vi "Mapping v10.6.0.vi"(5 "Simulate Spectra":bool, 7 "Simulate Drive":bool) -> ()   [LabVIEW 2010]
uses:
  TypeDefs/Mapping Spectra Params.ctl
  TypeDefs/Mapping Drive Params v10.6.0.ctl
  NPC3SG/TypeDefs/NPC3SG Set Positions.ctl
  NPC3SG/TypeDefs/NPC3SG Current Values.ctl
  iHR550/TypeDefs/iHR Current Values.ctl
  ITC503/TypeDefs/ITC503 Current Values.ctl
  TypeDefs/Mapping Input Parameters v10.6.0.ctl
  Symphony/TypeDefs/Symphony Area Format.ctl
  <vilib>/Utility/miscctls.llb/LVPointTypeDef.ctl
  Global Variables.vi
panel:
  in  "Input Parameters":T1={"Drive Connection Port"="", "ITC503 Current Values"={"ITC503 Heater"=0.0, "ITC503 Temperature"=0.0, "ITC503 P"=0.0, "ITC503 I"=0.0, "ITC503 D"=0.0, "ITC503 Setpoint"=0.0, "ITC503 Gradient"=0.0, "ITC503 Heater Auto"=FALSE, "ITC503 PID Auto"=FALSE}, "Wavelengths (nm)"=[], "Drive Current Values"={"Drive X Position"=0.0, "Drive Y Position"=0.0, "Drive Z Position"=0.0}, "iHR Current Values"={"iHR 550 Front Entrance"=0.0, "iHR550 Side Exit"=0.0, "iHR550 Wavelength"=897.9988, "iHR550 Exit Mirror"=2, "iHR550 Grating"="1", "Grating Index"=1}, "Spectra Settings"={"Integration Time"=1.0, "Repetitions"=1, "Mapping Spectra"=TRUE}, "CCD3500 Temperature"=0.0, "Simulate Drive"=FALSE, "Simulate Spectra"=FALSE, "JYCCDLib.IJYCCDReqd"=refnum, "CCD Area"={"XStart"=1, "YStart"=1, "XStop"=2048, "YStop"=512, "XBin"=1, "YBin"=1}, "CCD Gain"=1, "CCD ADC"=0} {"CCD ADC" items=["20 kHz       ", " 1 MHz       ", " 1 MHz Ultra ", "500 kHz Wrap"]; "CCD Gain" items=["High Light", "Best Dynamic Range", "High Sensitivity"]; "ITC503 Current Values"."ITC503 Gradient" format="%.2f"; "ITC503 Current Values"."ITC503 Setpoint" min=-273.0 max=300000.0 step=0.0001 format="%.1f"; "ITC503 Current Values"."ITC503 I" format="%_1f"; "ITC503 Current Values"."ITC503 P" format="%_1f"; "ITC503 Current Values"."ITC503 Temperature" min=0.0 max=1645.0 step=1e-05 format="%.2f"; "ITC503 Current Values"."ITC503 Heater" min=0.0 max=100.0 step=0.01 scale=0.0..100.0; "Drive Current Values"."Drive Z Position" min=-273.0 max=300000.0 step=0.0001 format="%.3f"; "Drive Current Values"."Drive Y Position" min=-273.0 max=300000.0 step=0.0001 format="%.3f"; "Drive Current Values"."Drive X Position" min=-273.0 max=300000.0 step=0.0001 format="%.3f"; "iHR Current Values"."iHR550 Exit Mirror" items=["EntranceMirror", "ExitMirror", "Front", "Side"]; "Spectra Settings"."Repetitions" min=1 max=100 step=1; "Spectra Settings"."Integration Time" min=0.5 max=6000.0 step=1.0 format="%.1f"}
  out "JYCCDLib.IJYCCDReqd":refnum<k7>
  out "AutoClose":bool
  out "ITC503 Temperature":dbl caption="Sample (K)" min=10.0 max=160.0 step=0.1 format="%.3f"
  out "CCD3500 Temperature":dbl caption="CCD (°C)" min=10.0 max=160.0 step=0.1 format="%.1f"
  in  "CCD Current Rep.":string="0/0"
  in  "Pause":bool
  out "Current Position":T3 {"Drive Z Position" min=-273.0 max=300000.0 step=0.0001 format="%.3f"; "Drive Y Position" min=-273.0 max=300000.0 step=0.0001 format="%.3f"; "Drive X Position" min=-273.0 max=300000.0 step=0.0001 format="%.3f"}
  out "Target Position":T7={"Drive X Set"=10.0, "Drive Y Set"=10.0, "Drive Z Set"=10.0} {"Drive X Set" min=10.0 max=160.0 step=0.1 format="%.3f"; "Drive Z Set" min=10.0 max=160.0 step=0.1 format="%.3f"; "Drive Y Set" min=10.0 max=160.0 step=0.1 format="%.3f"}
  out "Progress":u8(slide) max=10 scale=0.0..100.0
  out "Objective Running":bool caption="Obj."
  out "CCD Running":bool caption="CCD"
  in  "Save Map":bool
  in  "Spectra Params":T5={"Integration Time"=10.0, "Repetitions"=10, "Mapping Spectra"=TRUE} {"Repetitions" min=1 max=100 step=1; "Integration Time" min=0.5 max=6000.0 step=1.0 format="%.1f"}
  in  "Drive Settings":refnum<visa-resource-name>
  in  "Z Position":dbl caption="Z (µm)" min=0.0 max=100.0 step=0.1 format="%.1f"
  in  "Mapping Params":T8={"X Start Position"=0.0, "X Stop Position"=10.0, "Y Start Position"=0.0, "Y Stop Position"=10.0, "Step Size"=1.0} {"Step Size" min=0.005 max=20.0 step=0.005 format="%.3f"; "Y Stop Position" min=0.0 max=140.0 step=0.005 format="%.3f"; "Y Start Position" min=0.0 max=140.0 step=0.005 format="%.3f"; "X Stop Position" min=0.0 max=140.0 step=0.005 format="%.3f"; "X Start Position" min=0.0 max=140.0 step=0.005 format="%.3f"}
  in  "Exit":bool
  out "Measuring":bool
  in  "Start":bool
  out "Filename":string
  out "Full Data":dbl[][](array[numeric])
  out "Live Data":dbl[][](array[numeric])
  in  "ITC503 Current Values":T2 {"ITC503 Gradient" format="%.2f"; "ITC503 Setpoint" min=-273.0 max=300000.0 step=0.0001 format="%.1f"; "ITC503 I" format="%_1f"; "ITC503 P" format="%_1f"; "ITC503 Temperature" min=0.0 max=1645.0 step=1e-05 format="%.2f"; "ITC503 Heater" min=0.0 max=100.0 step=0.01 scale=0.0..100.0}
  in  "iHR Current Values":T4={"iHR 550 Front Entrance"=0.0, "iHR550 Side Exit"=0.0, "iHR550 Wavelength"=897.9988, "iHR550 Exit Mirror"=2, "iHR550 Grating"="1", "Grating Index"=1} {"iHR550 Exit Mirror" items=["EntranceMirror", "ExitMirror", "Front", "Side"]}
  in  "Wavelengths (nm)":dbl[](array[numeric])
  # "Status"
  # "Active"
  # "Target"
  # "Current"
  # "Parameters"
  # "Spectral"
  # "Spectral / Video Mapping"
  # "Mapping"
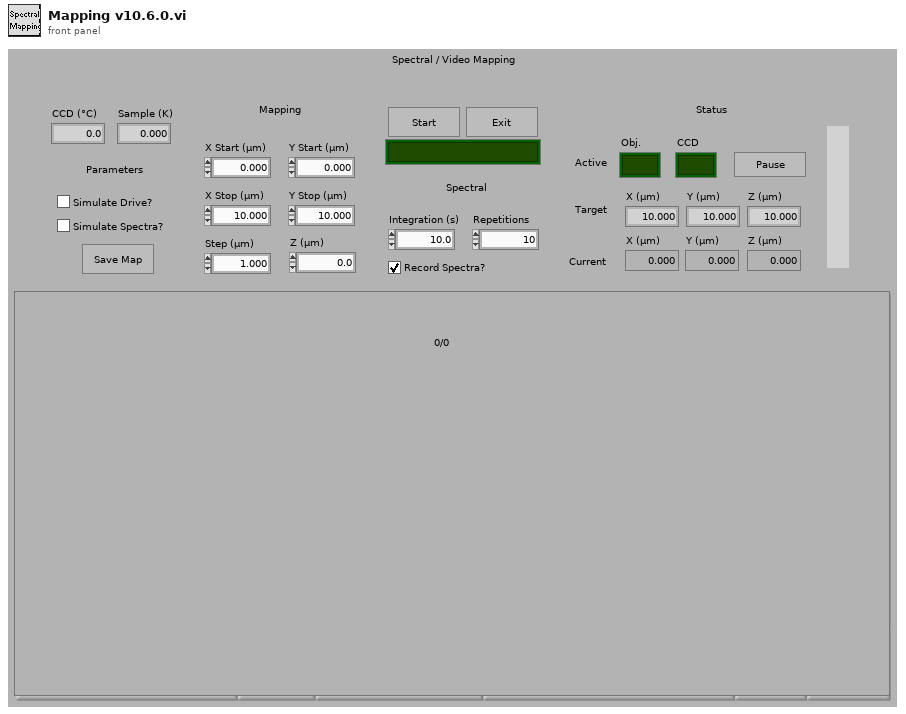
[diagram p1: front panel]
types:
  T1 = typedef "Mapping Input Parameters v10.6.0.ctl" = cluster{"Drive Connection Port":refnum<visa-resource-name>, "ITC503 Current Values":T2, "Wavelengths (nm)":dbl[], "Drive Current Values":T3, "iHR Current Values":T4, "Spectra Settings":T5, "CCD3500 Temperature":dbl, "Simulate Drive":bool, "Simulate Spectra":bool, "JYCCDLib.IJYCCDReqd":refnum<k7>, "CCD Area":T6, "CCD Gain":u16, "CCD ADC":u16}
  T2 = typedef "ITC503 Current Values.ctl" = cluster{"ITC503 Heater":dbl, "ITC503 Temperature":dbl, "ITC503 P":dbl, "ITC503 I":dbl, "ITC503 D":dbl, "ITC503 Setpoint":dbl, "ITC503 Gradient":dbl, "ITC503 Heater Auto":bool, "ITC503 PID Auto":bool}
  T3 = typedef "NPC3SG Current Values.ctl" = cluster{"Drive X Position":dbl, "Drive Y Position":dbl, "Drive Z Position":dbl}
  T4 = typedef "iHR Current Values.ctl" = cluster{"iHR 550 Front Entrance":dbl, "iHR550 Side Exit":dbl, "iHR550 Wavelength":dbl, "iHR550 Exit Mirror":i32, "iHR550 Grating":string, "Grating Index":i32}
  T5 = typedef "Mapping Spectra Params.ctl" = cluster{"Integration Time":dbl, "Repetitions":u16, "Mapping Spectra":bool}
  T6 = typedef "Symphony Area Format.ctl" = cluster{"XStart":i32, "YStart":i32, "XStop":i32, "YStop":i32, "XBin":i32, "YBin":i32}
  T7 = typedef "NPC3SG Set Positions.ctl" = cluster{"Drive X Set":dbl, "Drive Y Set":dbl, "Drive Z Set":dbl}
  T8 = typedef "Mapping Drive Params v10.6.0.ctl" = cluster{"X Start Position":dbl, "X Stop Position":dbl, "Y Start Position":dbl, "Y Stop Position":dbl, "Step Size":dbl}
  T9 = typedef "LVPointTypeDef.ctl" = cluster{"Horizontal":i16, "Vertical":i16}
  T10 = cluster{"Intensities":dbl[], "Wavelengths":dbl[]}[]
  T11 = cluster{"Intensities":dbl[], "Wavelengths":dbl[]}
  T12 = enum32{"invalid app kind", "Development System", "Run Time System", "Student Edition", "Embedded LabVIEW", "Evaluation", "Custom"}
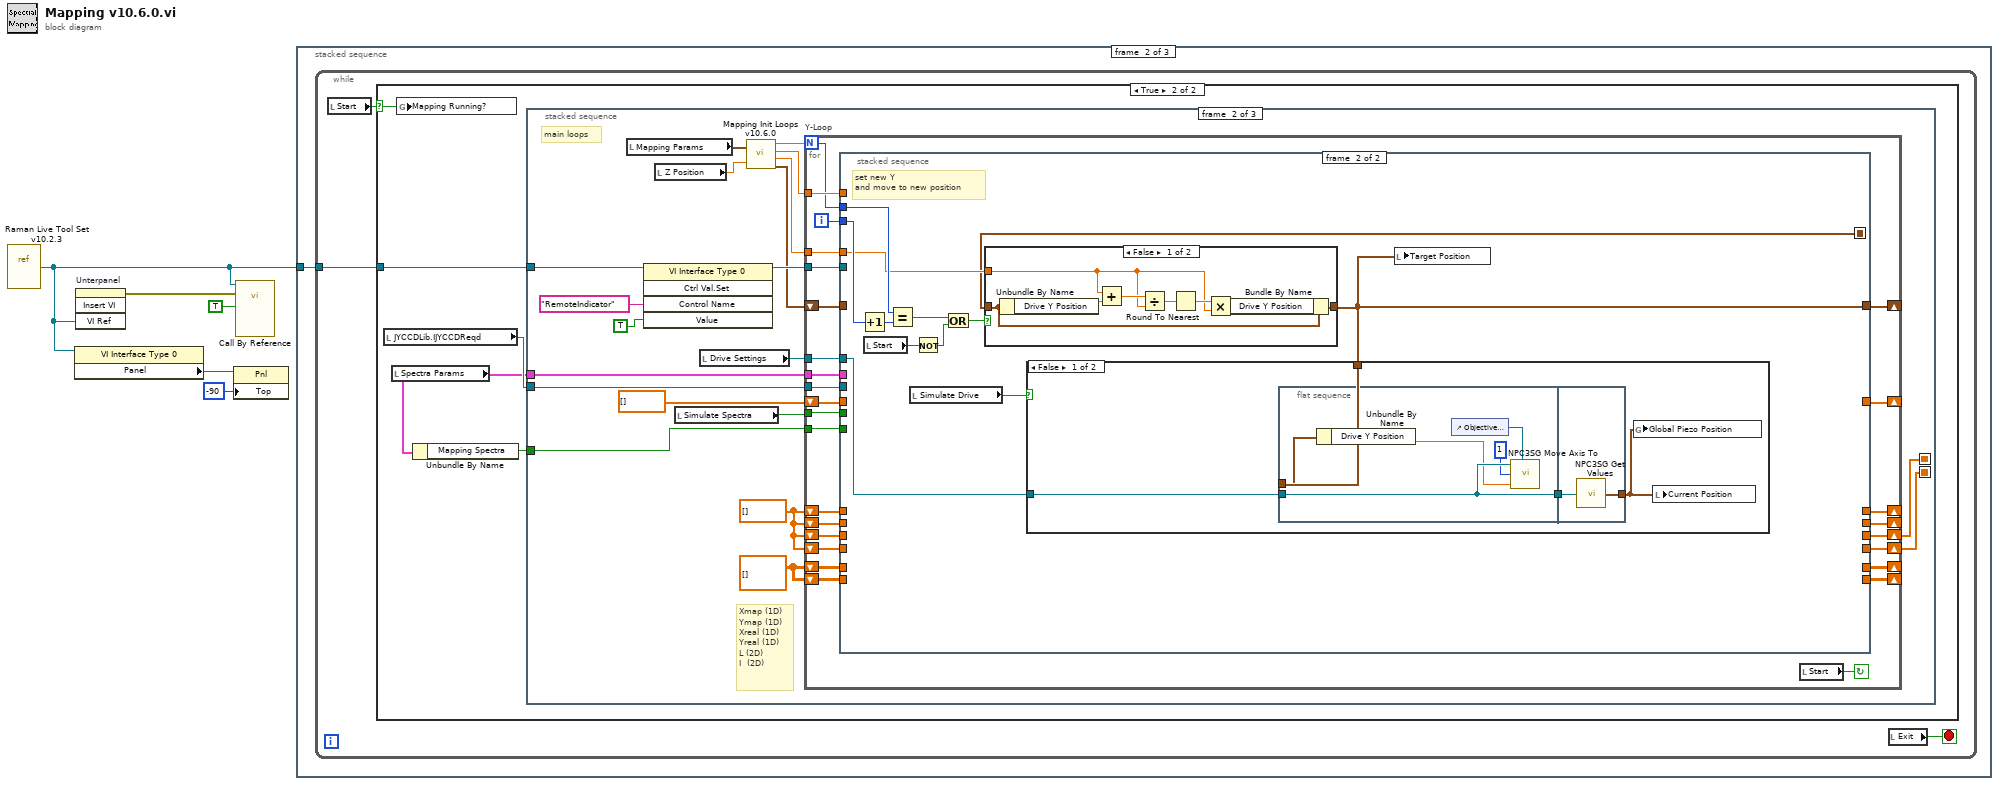
[diagram p0: block diagram]
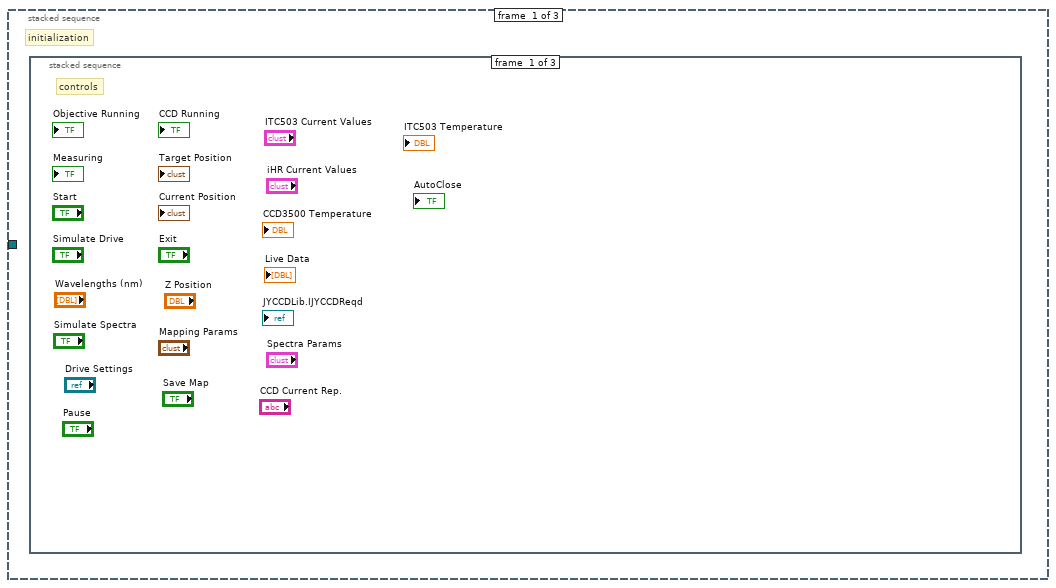
[diagram p2: hidden frame]
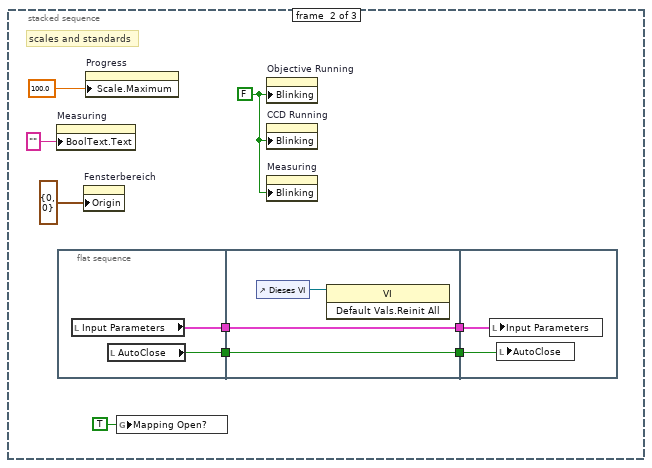
[diagram p3: hidden frame]
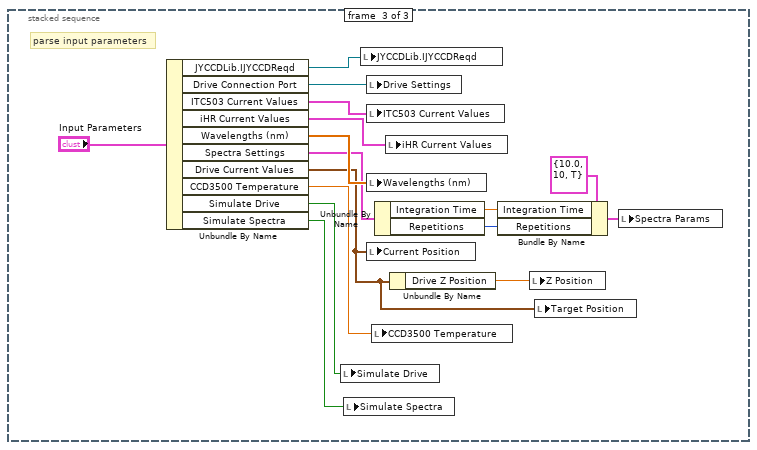
[diagram p4: hidden frame]
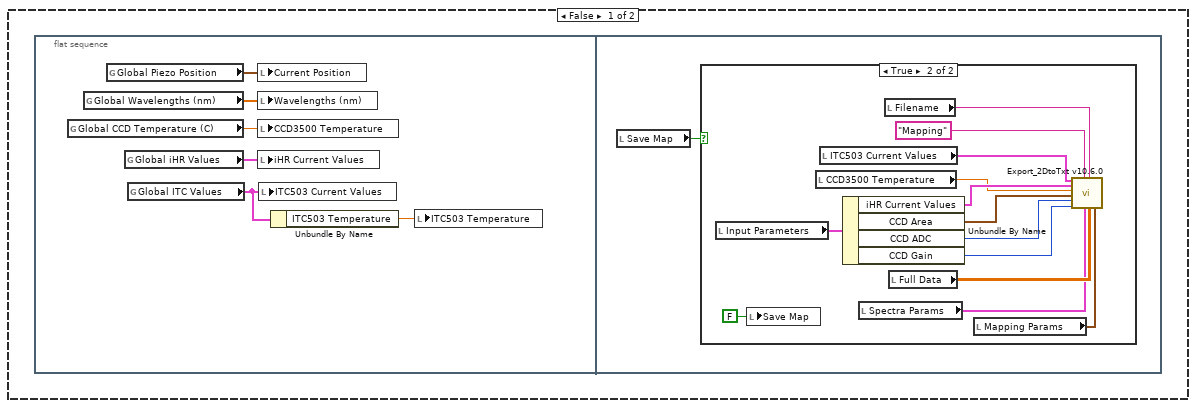
[diagram p5: hidden frame]
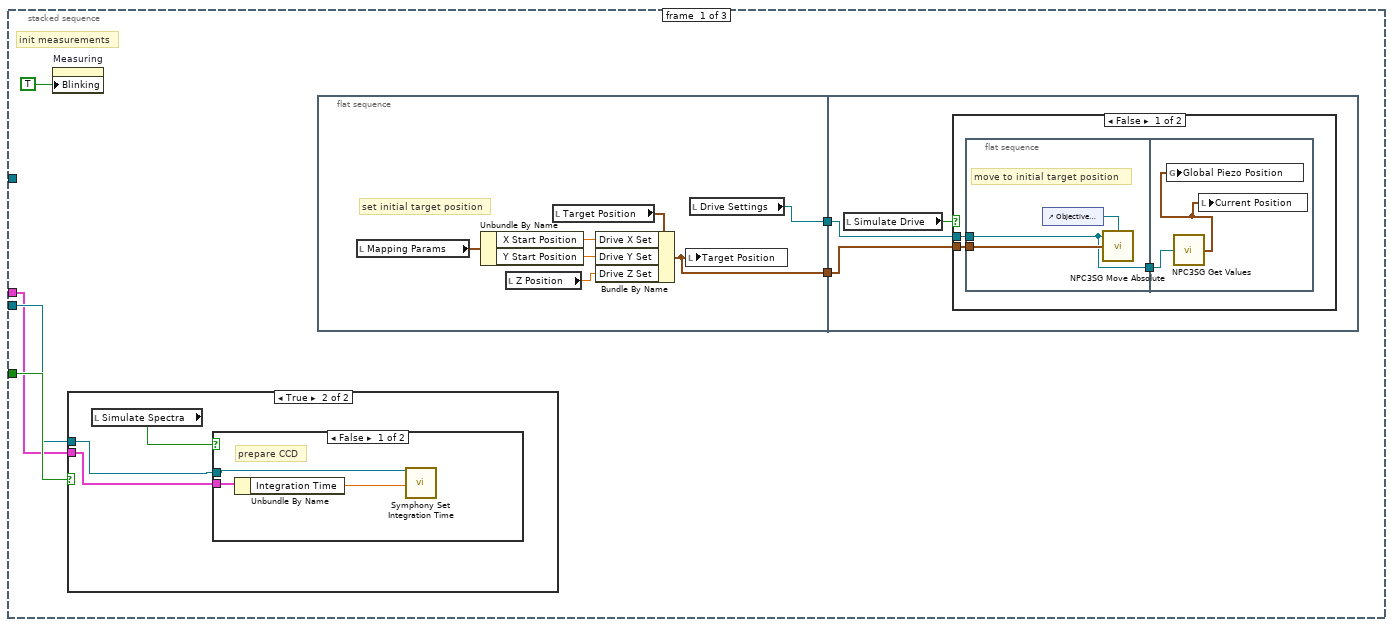
[diagram p7: hidden frame]
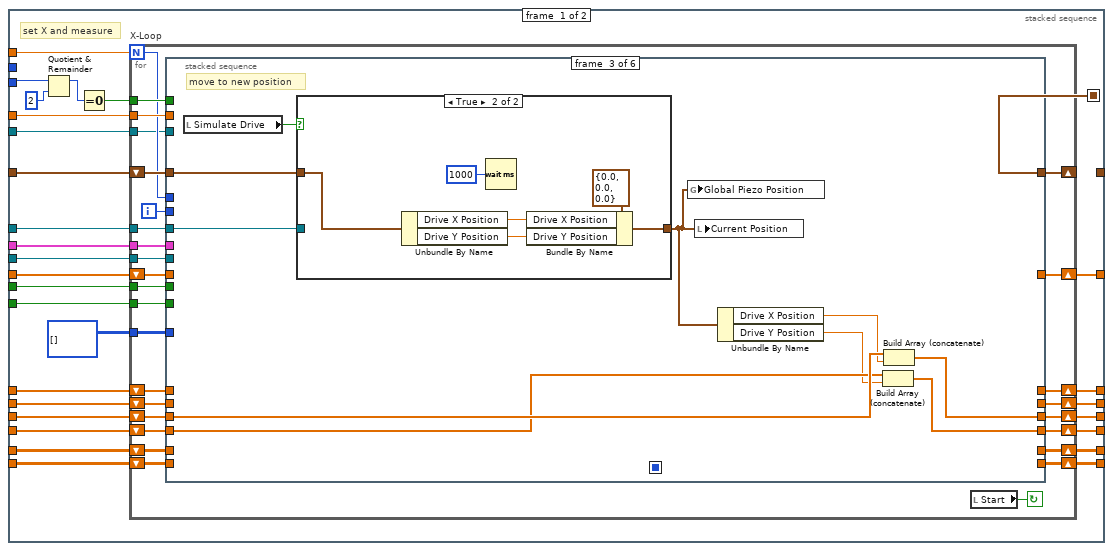
[diagram p11: hidden frame]
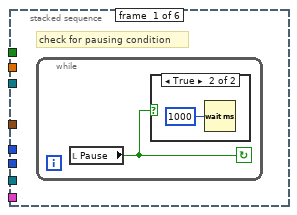
[diagram p12: hidden frame]
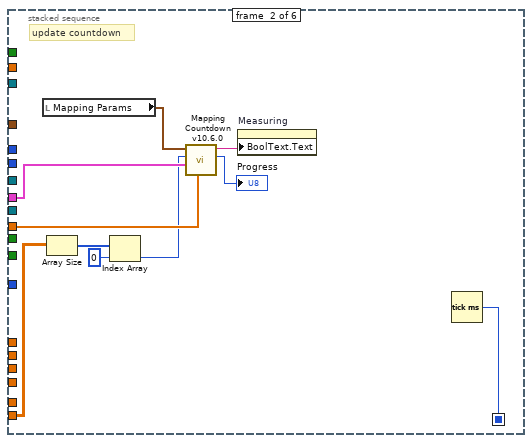
[diagram p14: hidden frame]
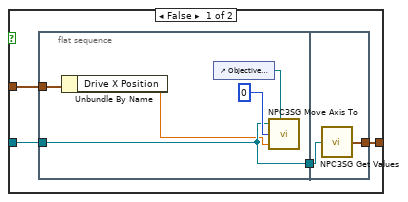
[diagram p15: hidden frame]
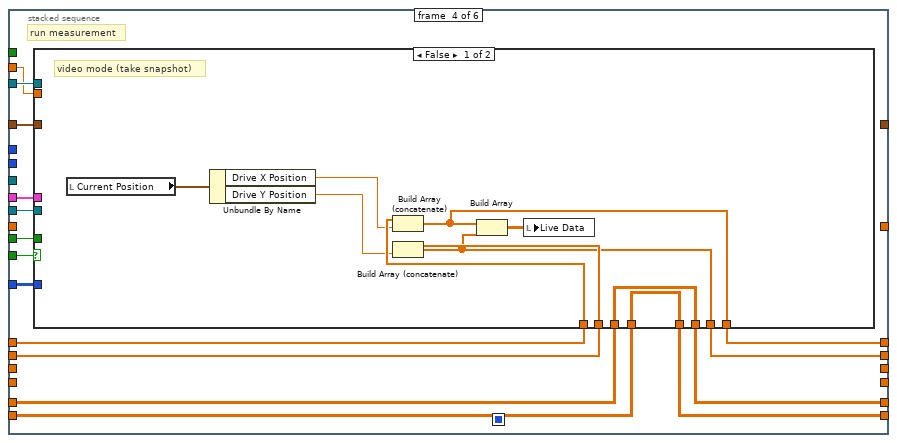
[diagram p16: hidden frame]
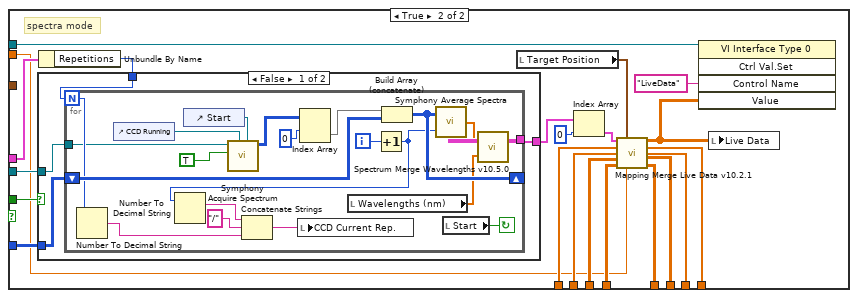
[diagram p17: hidden frame]
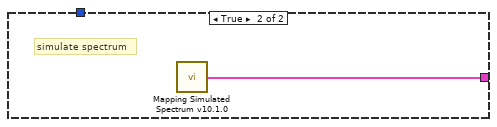
[diagram p18: hidden frame]
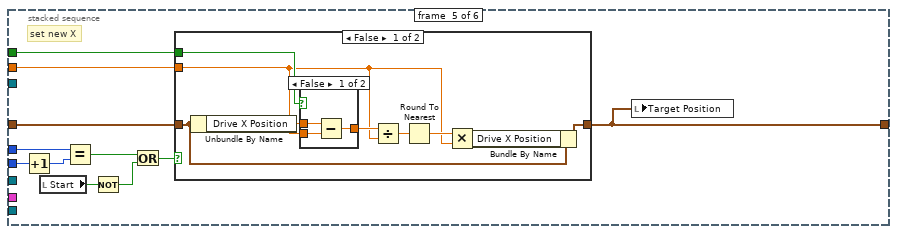
[diagram p19: hidden frame]
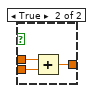
[diagram p20: hidden frame]
diagram:
  n1 = vi-ref "Raman Live Tool Set v10.2.3.vi"() -> (w3:refnum<vi>)
  n2 = property class="VI Interface Type 0"(reference=w3) -> ("Panel"=w2:refnum<vi>)  [unwired: 1 in, 2 out]
  n3 = invoke on="Unterpanel" class="Unterpanel" method="Insert VI"("VI Ref"=w3) -> (error out=w5:errorcluster)  [unwired: 3 in, 3 out]
  n4 = property class="Pnl"(reference=w2, "Top"=-90 ("Position:Oben")) -> ()  [unwired: 1 in, 2 out]
  n5 = call-by-ref "?"(reference=w3, error in=w5, "RemoteIndicator"=TRUE) -> ()  [unwired: 3 in, 2 out]
  n6 = stacked-sequence {
    tunnel: w3 -> [_ w38 w404]
    frame #0 {
      # "initialization"
      n7 = stacked-sequence {
        frame #0 {
          # "controls"
        }
        frame #1 {
          w12 = FALSE ("Blinkend")
          # "scales and standards"
          n8 = property on="Measuring" class="Bool (strict)"("BoolText.Text"="" ("Boolescher Text.Text")) -> ()  [unwired: 2 in, 2 out]
          n9 = flat-sequence {
            tunnel: [w16] -> w9
            tunnel: [w15] -> w6
            tunnel: [w18] -> w10
            tunnel: w9 -> [w18]
            tunnel: [w17] -> w7
            tunnel: w6 -> [w17]
            tunnel: w10 -> [w21]
            tunnel: w7 -> [w20]
            frame #0 {
              n10 = local read "Input Parameters"() -> (w16:T1)
              n11 = local read "AutoClose"() -> (w15:bool)
            }
            frame #1 {
              n12 = control-ref of="Dieses VI"() -> (w19:refnum<vi>)
              n13 = invoke class="VI" method="Default Vals.Reinit All"(reference=w19) -> ()  [unwired: 2 in, 3 out]
            }
            frame #2 {
              n14 = local write "Input Parameters"(w21) -> ()
              n15 = local write "AutoClose"(w20) -> ()
            }
          }
          n16 = property on="Fensterbereich" class="Pane"("Origin"=T9 {"Horizontal"=0, "Vertical"=0}) -> ()  [unwired: 2 in, 2 out]
          n17 = property on="Progress" class="Slide (strict)"("Scale.Maximum"=100.0 ("Skalierung.Bereich:Maximum")) -> ()  [unwired: 2 in, 2 out]
          n18 = global write "Global Variables.vi" "Mapping Open?"(TRUE ("Mapping Open?")) -> ()
          n19 = property on="Objective Running" class="Bool (strict)"("Blinking"=w12) -> ()  [unwired: 2 in, 2 out]
          n20 = property on="CCD Running" class="Bool (strict)"("Blinking"=w12) -> ()  [unwired: 2 in, 2 out]
          n21 = property on="Measuring" class="Bool (strict)"("Blinking"=w12) -> ()  [unwired: 2 in, 2 out]
        }
        frame #2 {
          # "parse input parameters"
          n22 = Unbundle By Name("Input Parameters") -> ("JYCCDLib.IJYCCDReqd"=w24:refnum<k7>, "Drive Connection Port"=w36:refnum<visa-resource-name>, "ITC503 Current Values"=w37:T2, "iHR Current Values"=w27:T4, "Wavelengths (nm)"=w35:dbl[], "Spectra Settings"=w33:T5, "Drive Current Values"=w22:T3, "CCD3500 Temperature"=w28:dbl, "Simulate Drive"=w26:bool, "Simulate Spectra"=w25:bool)
          n23 = local write "Simulate Drive"(w26) -> ()
          n24 = local write "Simulate Spectra"(w25) -> ()
          n25 = local write "JYCCDLib.IJYCCDReqd"(w24) -> ()
          n26 = local write "Drive Settings"(w36) -> ()
          n27 = local write "ITC503 Current Values"(w37) -> ()
          n28 = local write "Wavelengths (nm)"(w35) -> ()
          n29 = local write "Current Position"(w22) -> ()
          n30 = local write "CCD3500 Temperature"(w28) -> ()
          n31 = Unbundle By Name(w33) -> ("Integration Time"=w31:dbl, "Repetitions"=w30:u16)
          n32 = local write "iHR Current Values"(w27) -> ()
          n33 = Unbundle By Name(w22) -> ("Drive Z Position"=w34:dbl)
          n34 = Bundle By Name(cluster=T5 {"Integration Time"=10.0, "Repetitions"=10, "Mapping Spectra"=TRUE} ("Mapping Spectra Settings"), "Integration Time"=w31, "Repetitions"=w30) -> (w29:T5)
          n35 = local write "Z Position"(w34) -> ()
          n36 = local write "Target Position"(w22) -> ()
          n37 = local write "Spectra Params"(w29) -> ()
        }
      }
    }
    frame #1 {
      n38 = while {
        tunnel: w38 -> [w41]
        stop <- w40 stop-if-true
        n39 = local read "Start"() -> (w39:bool)
        n40 = case shown="True" w39 {
          selector: w39 -> [_ w62]
          tunnel: w41 -> [_ w66]
          frame False {
            n41 = flat-sequence {
              frame #0 {
                n42 = global read "Global Variables.vi" "Global CCD Temperature (C)"() -> (w47:dbl)
                n43 = global read "Global Variables.vi" "Global Wavelengths (nm)"() -> (w45:dbl[])
                n44 = global read "Global Variables.vi" "Global Piezo Position"() -> (w46:T3)
                n45 = global read "Global Variables.vi" "Global iHR Values"() -> (w44:T4)
                n46 = global read "Global Variables.vi" "Global ITC Values"() -> (w43:T2)
                n47 = local write "Current Position"(w46) -> ()
                n48 = local write "Wavelengths (nm)"(w45) -> ()
                n49 = local write "CCD3500 Temperature"(w47) -> ()
                n50 = local write "iHR Current Values"(w44) -> ()
                n51 = local write "ITC503 Current Values"(w43) -> ()
                n52 = Unbundle By Name(w43) -> ("ITC503 Temperature"=w42:dbl)
                n53 = local write "ITC503 Temperature"(w42) -> ()
              }
              frame #1 {
                n54 = local read "Save Map"() -> (w48:bool)
                n55 = case shown="True" w48 {
                  frame False {
                  }
                  frame True {
                    n56 = local read "Input Parameters"() -> (w57:T1)
                    n57 = local write "Save Map"(FALSE ("Save Map")) -> ()
                    n58 = local read "CCD3500 Temperature"() -> (w51:dbl)
                    n59 = local read "ITC503 Current Values"() -> (w54:T2)
                    n60 = Unbundle By Name(w57) -> ("iHR Current Values"=w52:T4, "CCD Area"=w53:T6, "CCD ADC"=w56:u16, "CCD Gain"=w55:u16)
                    n61 = local read "Spectra Params"() -> (w50:T5)
                    n62 = local read "Filename"() -> (w60:string)
                    n63 = local read "Full Data"() -> (w58:dbl[][])
                    n64 = local read "Mapping Params"() -> (w49:T8)
                    n65 = call "Export_2DtoTxt v10.6.0.vi"("ITC503 Current Values"=w54, "iHR Current Values"=w52, "CCD Temperature"=w51, "CCD Area"=w53, "CCD ADC"=w56, "CCD Gain"=w55, "Export Type"="Mapping", "Spectra Settings"=w50, "Filename"=w60, "Data (2D)"=w58, "Mapping Parameters"=w49) -> ()  [unwired: 8 in, 1 out]
                  }
                }
              }
            }
          }
          frame True {
            n66 = local read "JYCCDLib.IJYCCDReqd"() -> (w64:refnum<k7>)
            n67 = local read "Spectra Params"() -> (w63:T5)
            n68 = global write "Global Variables.vi" "Mapping Running?"(w62) -> ()
            n69 = Unbundle By Name(w63) -> ("Mapping Spectra"=w65:bool)
            n70 = stacked-sequence {
              seq-local: [_ w97 _] -> [_ _ w379]
              seq-local: [_ w98 _] -> [_ _ w378]
              tunnel: w66 -> [_ w108 _]
              tunnel: w65 -> [w71 w107 w380]
              tunnel: w63 -> [w69 w105 _]
              tunnel: w64 -> [w70 w104 _]
              frame #0 {
                # "init measurements"
                n71 = property on="Measuring" class="Bool (strict)"("Blinking"=TRUE ("Blinkend")) -> ()  [unwired: 2 in, 2 out]
                n72 = case shown="True" w71 {
                  tunnel: w70 -> [_ w93]
                  tunnel: w69 -> [_ w92]
                  frame False {
                  }
                  frame True {
                    n73 = local read "Simulate Spectra"() -> (w91:bool)
                    n74 = case shown="False" w91 {
                      tunnel: w93 -> [w96 _]
                      tunnel: w92 -> [w95 _]
                      frame False {
                        # "prepare CCD"
                        n75 = Unbundle By Name(w95) -> ("Integration Time"=w94:dbl)
                        n76 = call "Symphony Set Integration Time.vi"("JYCCDLib.IJYCCDReqd"=w96, "Integration (s)"=w94) -> ()  [unwired: 13 in, 1 out]
                      }
                      frame True {
                      }
                    }
                  }
                }
                n77 = flat-sequence {
                  tunnel: [w74] -> w68
                  tunnel: [w73] -> w67
                  tunnel: w68 -> [w80]
                  tunnel: w67 -> [w81]
                  frame #0 {
                    # "set initial target position"
                    n78 = local read "Mapping Params"() -> (w79:T8)
                    n79 = Unbundle By Name(w79) -> ("X Start Position"=w77:dbl, "Y Start Position"=w76:dbl)
                    n80 = local read "Z Position"() -> (w75:dbl)
                    n81 = local read "Target Position"() -> (w78:T7)
                    n82 = Bundle By Name(cluster=w78, "Drive X Set"=w77, "Drive Y Set"=w76, "Drive Z Set"=w75) -> (w74:T7)
                    n83 = local write "Target Position"(w74) -> ()
                    n84 = local read "Drive Settings"() -> (w73:refnum<visa-resource-name>)
                  }
                  frame #1 {
                    n85 = local read "Simulate Drive"() -> (w82:bool)
                    n86 = case shown="False" w82 {
                      tunnel: w81 -> [w85 _]
                      tunnel: w80 -> [w83 _]
                      frame False {
                        n87 = flat-sequence {
                          tunnel: w85 -> [w86]
                          tunnel: [w86] -> w84
                          tunnel: w83 -> [w87]
                          tunnel: w84 -> [w89]
                          frame #0 {
                            # "move to initial target position"
                            n88 = control-ref of="Objective Running"() -> (w88:refnum<vi>)
                            n89 = call "NPC3SG Move Absolute.vi"("Running"=w88, "Drive New Abs. Positions"=w87, "Drive Visa Name"=w86) -> ()  [unwired: 2 in]
                          }
                          frame #1 {
                            n90 = call "NPC3SG Get Values.vi"("Drive Visa Name"=w89) -> ("Drive Current Values"=w90:T3)
                            n91 = global write "Global Variables.vi" "Global Piezo Position"(w90) -> ()
                            n92 = local write "Current Position"(w90) -> ()
                          }
                        }
                      }
                      frame True {
                      }
                    }
                  }
                }
              }
              frame #1 {
                w116 = dbl[][] []
                w99 = dbl[] []
                # "main loops"
                # "Xmap (1D)\nYmap (1D)\nXreal (1D)\nYreal (1D)\nL (2D)\nI  (2D)"
                n93 = local read "Mapping Params"() -> (w102:T8)
                n94 = invoke class="VI Interface Type 0" method="Ctrl Val.Set"(reference=w108, "Control Name"="RemoteIndicator" ("Elementname"), "Value"=TRUE) -> (reference out=w110:refnum<vi>)  [unwired: 2 in, 4 out]
                n95 = local read "Z Position"() -> (w101:dbl)
                n96 = local read "Simulate Spectra"() -> (w100:bool)
                n97 = local read "Drive Settings"() -> (w103:refnum<visa-resource-name>)
                n98 = call "Mapping Init Loops v10.6.0.vi"("Z Position"=w101, "Mapping Params"=w102) -> ("Start Positions"=w109:T3, "Step Size"=w111:dbl, "X Steps"=w112:dbl, "Y Steps"=w113:dbl)
                n99 = for "Y-Loop" {
                  N: w113 -> [w129]
                  tunnel: w112 -> [w142]
                  tunnel: w111 -> [w141]
                  shift-right: [w127] -> _
                  shift-left: w109 -> [w128]
                  shift-right: [w133] -> _
                  shift-left: w116 -> [w137]
                  shift-right: [w134] -> _
                  shift-left: w116 -> [w138]
                  shift-right: [w136] -> _
                  shift-left: w99 -> [w140]
                  shift-right: [w135] -> _
                  shift-left: w99 -> [w139]
                  tunnel: w110 -> [w131]
                  tunnel: w100 -> [w130]
                  tunnel: w103 -> [w126]
                  tunnel: w107 -> [w125]
                  tunnel: w105 -> [w124]
                  shift-right: [w122] -> _
                  shift-left: dbl[] [] -> [w123]
                  tunnel: w104 -> [w121]
                  shift-right: [w118] -> w98
                  shift-left: w99 -> [w119]
                  shift-right: [w117] -> w97
                  shift-left: w99 -> [w120]
                  i -> [w132]
                  stop <- w143 continue-if-true
                  n100 = stacked-sequence {
                    seq-local: [w157 _] -> [_ w353]
                    tunnel: w142 -> [w172 _]
                    tunnel: w141 -> [w171 w354]
                    tunnel: w140 -> [w170 _]
                    tunnel: w139 -> [w169 _]
                    tunnel: w138 -> [w168 _]
                    tunnel: w137 -> [w144 _]
                    tunnel: [w167 _] -> w136
                    tunnel: [w166 _] -> w135
                    tunnel: [w165 _] -> w134
                    tunnel: [w164 _] -> w133
                    tunnel: w132 -> [w161 w357]
                    tunnel: w131 -> [w159 _]
                    tunnel: w130 -> [w158 _]
                    tunnel: w129 -> [_ w355]
                    tunnel: w128 -> [w156 _]
                    tunnel: [_ w351] -> w127
                    tunnel: w126 -> [w155 w352]
                    tunnel: w125 -> [w154 _]
                    tunnel: w124 -> [w153 _]
                    tunnel: w123 -> [w152 _]
                    tunnel: [w151 _] -> w122
                    tunnel: w121 -> [w150 _]
                    tunnel: w120 -> [w148 _]
                    tunnel: w119 -> [w147 _]
                    tunnel: [w146 _] -> w118
                    tunnel: [w145 _] -> w117
                    frame #0 {
                      # "set X and measure"
                      n101 = Quotient & Remainder(x=w161, y=2) -> (x-y*floor(x/y)=w162:i32)  [unwired: 1 out]
                      n102 = Equal To 0?(x=w162) -> (x = 0?=w160:bool)
                      n103 = for "X-Loop" {
                        N: w172 -> [w186]
                        tunnel: w171 -> [w198]
                        shift-right: [w197] -> w157
                        shift-left: w156 -> [w199]
                        shift-right: [w192] -> w167
                        shift-left: w170 -> [w196]
                        shift-right: [w191] -> w166
                        shift-left: w169 -> [w195]
                        shift-right: [w189] -> w165
                        shift-left: w168 -> [w194]
                        shift-right: [w190] -> w164
                        shift-left: w144 -> [w193]
                        tunnel: w160 -> [w188]
                        tunnel: w159 -> [w185]
                        tunnel: w158 -> [w184]
                        tunnel: w155 -> [w183]
                        tunnel: w154 -> [w182]
                        tunnel: w153 -> [w181]
                        shift-right: [w180] -> w151
                        shift-left: w152 -> [w179]
                        tunnel: w150 -> [w178]
                        tunnel: u16[][] [] -> [w177]
                        shift-right: [w173] -> w145
                        shift-left: w148 -> [w176]
                        shift-right: [w174] -> w146
                        shift-left: w147 -> [w175]
                        i -> [w187]
                        stop <- w200 continue-if-true
                        n104 = stacked-sequence {
                          seq-local: [_ w207 _ _ _ _] -> [_ _ _ _ _ w342]
                          tunnel: w199 -> [_ _ w222 w255 w319 _]
                          tunnel: w198 -> [_ _ _ w240 w317 _]
                          tunnel: [_ _ _ _ w316 _] -> w197
                          tunnel: w196 -> [_ _ _ w254 _ _]
                          tunnel: w195 -> [_ _ _ w253 _ _]
                          tunnel: w194 -> [_ _ _ w251 _ _]
                          tunnel: w193 -> [_ w206 _ w252 _ _]
                          tunnel: [_ _ _ w250 _ _] -> w192
                          tunnel: [_ _ _ w249 _ _] -> w191
                          tunnel: [_ _ _ w248 _ _] -> w190
                          tunnel: [_ _ _ w247 _ _] -> w189
                          tunnel: w188 -> [_ _ _ _ w318 _]
                          tunnel: w187 -> [_ _ _ _ w322 _]
                          tunnel: w186 -> [_ _ _ _ w320 _]
                          tunnel: w185 -> [_ _ _ w246 _ _]
                          tunnel: w184 -> [_ _ _ w245 _ _]
                          tunnel: w183 -> [_ _ w220 _ _ _]
                          tunnel: w182 -> [_ _ _ w244 _ _]
                          tunnel: w181 -> [_ w209 _ w242 _ _]
                          tunnel: [_ _ _ _ _ w339] -> w180
                          tunnel: w179 -> [_ w208 _ _ _ w341]
                          tunnel: w178 -> [_ _ _ w243 _ _]
                          tunnel: w177 -> [_ _ _ w241 _ _]
                          tunnel: w176 -> [_ _ w219 _ _ _]
                          tunnel: w175 -> [_ _ w218 _ _ _]
                          tunnel: [_ _ w215 _ _ _] -> w174
                          tunnel: [_ _ w214 _ _ _] -> w173
                          frame #0 {
                            # "check for pausing condition"
                            n105 = while {
                              stop <- w201 continue-if-true
                              n106 = local read "Pause"() -> (w201:bool)
                              n107 = case shown="True" w201 {
                                frame False {
                                }
                                frame True {
                                n108 = Wait (ms)(milliseconds to wait=u32 1000) -> ()  [unwired: 1 out]
                                }
                              }
                            }
                          }
                          frame #1 {
                            # "update countdown"
                            n109 = local read "Mapping Params"() -> (w212:T8)
                            n110 = Array Size(array=w206) -> (size(s)=w205:i32[])
                            n111 = Index Array(array=w205, index=0) -> (element=w203:i32)
                            n112 = call "Mapping Countdown v10.6.0.vi"("Execution Times (s)"=w208, "Mapping Spectra Settings"=w209, "Ready Steps"=w203, "Mapping Drive Parameters"=w212) -> ("Progress"=→"Progress":i16, "Time String"=w210:string)  [unwired: 6 in]
                            n113 = property on="Measuring" class="Bool (strict)"("BoolText.Text"=w210) -> ()  [unwired: 2 in, 2 out]
                            n114 = Tick Count (ms)() -> (millisecond timer value=w207:u32)
                          }
                          frame #2 {
                            # "move to new position"
                            n115 = local read "Simulate Drive"() -> (w221:bool)
                            n116 = case shown="True" w221 {
                              tunnel: w222 -> [w226 w238]
                              tunnel: w220 -> [w225 _]
                              tunnel: [w223 w234] -> w213
                              frame False {
                                n117 = flat-sequence {
                                tunnel: w226 -> [w228]
                                tunnel: w225 -> [w229]
                                tunnel: [w229] -> w224
                                tunnel: w224 -> [w233]
                                tunnel: [w232] -> w223
                                frame #0 {
                                n118 = Unbundle By Name(w228) -> ("Drive X Position"=w227:dbl)
                                n119 = control-ref of="Objective Running"() -> (w230:refnum<vi>)
                                n120 = call "NPC3SG Move Axis To.vi"("Drive Visa Name"=w229, "Running"=w230, "Axis"=0, "Drive Set"=w227) -> ()  [unwired: 3 in, 1 out]
                                }
                                frame #1 {
                                n121 = call "NPC3SG Get Values.vi"("Drive Visa Name"=w233) -> ("Drive Current Values"=w232:T3)
                                }
                                }
                              }
                              frame True {
                                n122 = Unbundle By Name(w238) -> ("Drive X Position"=w239:dbl, "Drive Y Position"=w236:dbl)
                                n123 = Wait (ms)(milliseconds to wait=u32 1000 ("Zu wartende ms")) -> ()  [unwired: 1 out]
                                n124 = Bundle By Name(cluster=T3 {"Drive X Position"=0.0, "Drive Y Position"=0.0, "Drive Z Position"=0.0} ("Drive Current Values"), "Drive X Position"=w239, "Drive Y Position"=w236) -> (w234:T3)
                              }
                            }
                            n125 = global write "Global Variables.vi" "Global Piezo Position"(w213) -> ()
                            n126 = local write "Current Position"(w213) -> ()
                            n127 = Unbundle By Name(w213) -> ("Drive X Position"=w217:dbl, "Drive Y Position"=w216:dbl)
                            n128 = Build Array (concatenate)(w218, w216) -> (w215:dbl[])
                            n129 = Build Array (concatenate)(w219, w217) -> (w214:dbl[])
                          }
                          frame #3 {
                            # "run measurement"
                            n130 = case shown="False" w244 {
                              tunnel: w255 -> [_ _]
                              tunnel: w254 -> [w262 w283]
                              tunnel: w253 -> [w261 w282]
                              tunnel: w252 -> [w264 w280]
                              tunnel: w251 -> [w265 w281]
                              tunnel: [w259 w277] -> w250
                              tunnel: [w260 w276] -> w249
                              tunnel: [w264 w279] -> w248
                              tunnel: [w265 w278] -> w247
                              tunnel: w246 -> [_ w285]
                              tunnel: w245 -> [_ w284]
                              tunnel: w243 -> [_ w273]
                              tunnel: w242 -> [_ w272]
                              tunnel: w241 -> [_ w270]
                              tunnel: w240 -> [_ w266]
                              frame False {
                                # "video mode (take snapshot)"
                                n131 = local read "Current Position"() -> (w263:T3)
                                n132 = Unbundle By Name(w263) -> ("Drive X Position"=w258:dbl, "Drive Y Position"=w257:dbl)
                                n133 = Build Array (concatenate)(w262, w258) -> (w259:dbl[])
                                n134 = Build Array (concatenate)(w261, w257) -> (w260:dbl[])
                                n135 = Build Array(w259, w260) -> (w256:dbl[][])
                                n136 = local write "Live Data"(w256) -> ()
                              }
                              frame True {
                                # "spectra mode"
                                n137 = Unbundle By Name(w272) -> ("Repetitions"=w271:u16)
                                n138 = case shown="False" w284 {
                                tunnel: [w289 w311] -> w269
                                tunnel: w273 -> [w290 _]
                                tunnel: w271 -> [w288 _]
                                tunnel: w270 -> [w287 _]
                                frame False {
                                n139 = for {
                                N: w288 -> [w297]
                                shift-right: [w308] -> _
                                shift-left: w287 -> [w309]
                                tunnel: [w306] -> w289
                                tunnel: w290 -> [w295]
                                i -> [w310]
                                stop <- w304 continue-if-true
                                n140 = Number To Decimal String(number=w297) -> (decimal integer string=w300:string)  [unwired: 1 in]
                                n141 = control-ref of="CCD Running"() -> (w303:refnum<vi>)
                                n142 = control-ref of="Start"() -> (w302:refnum<vi>)
                                n143 = call "Symphony Acquire Spectrum.vi"("Acquire"=w302, "Running"=w303, "ShutterOpen"=TRUE, "JYCCDLib.IJYCCDReqd"=w295) -> ("Raw Data"=w292:i32[][])  [unwired: 6 in, 1 out]
                                n144 = Index Array(array=w292, index (row)=0) -> (element=w291:i32[])  [unwired: 1 in]
                                n145 = local read "Wavelengths (nm)"() -> (w305:dbl[])
                                n146 = Increment(x=w310) -> (x+1=w296:i32)
                                n147 = Number To Decimal String(number=w296) -> (decimal integer string=w299:string)  [unwired: 1 in]
                                n148 = Concatenate Strings(w299, "/" ("string"), w300) -> (w298:string)
                                n149 = local write "CCD Current Rep."(w298) -> ()
                                n150 = Build Array (concatenate)(w291, w309) -> (w308:i32[][])
                                n151 = call "Symphony Average Spectra.vi"("Repetitions"=w296, "Raw Spectra"=w308) -> ("Raw Spectrum"=w307:dbl[])
                                n152 = local read "Start"() -> (w304:bool)
                                n153 = call "Spectrum Merge Wavelengths v10.5.0.vi"("Wavelengths (nm)"=w305, "Raw Spectrum"=w307) -> ("Spectrum-Cluster"=w306:T10)  [unwired: 1 out]
                                }
                                }
                                frame True {
                                # "simulate spectrum"
                                n154 = call "Mapping Simulated Spectrum v10.1.0.vi"() -> ("Simulated Spectrum"=w311:cluster{i32[], dbl[]}[])
                                }
                                }
                                n155 = local read "Target Position"() -> (w275:T7)
                                n156 = Index Array(array=w269, index=0 ("Index")) -> (element=w268:T11)
                                n157 = call "Mapping Merge Live Data v10.2.1.vi"("New Spectrum"=w268, "Target Position"=w275, "X in (1D)"=w283, "Y in (1D)"=w282, "L in (2D)"=w281, "I in (2D)"=w280, "Step Size"=w266) -> ("Live Data"=w274:dbl[][], "X out (1D)"=w277:dbl[], "Y out (1D)"=w276:dbl[], "L out (2D)"=w278:dbl[][], "I out (2D)"=w279:dbl[][])  [unwired: 4 in]
                                n158 = invoke class="VI Interface Type 0" method="Ctrl Val.Set"(reference=w285, "Control Name"="LiveData" ("Elementname"), "Value"=w274) -> ()  [unwired: 2 in, 5 out]
                                n159 = local write "Live Data"(w274) -> ()
                              }
                            }
                          }
                          frame #4 {
                            # "set new X"
                            n160 = Increment(x=w322) -> (x+1=w321:i32)
                            n161 = local read "Start"() -> (w315:bool)
                            n162 = Equal?(x=w320, y=w321) -> (x = y?=w312:bool)
                            n163 = Not(x=w315) -> (.not. x?=w314:bool)
                            n164 = Or(x=w312, y=w314) -> (x .or. y?=w313:bool)
                            n165 = case shown="False" w313 {
                              tunnel: w319 -> [w330 w338]
                              tunnel: [w329 w338] -> w316
                              tunnel: w318 -> [w328 _]
                              tunnel: w317 -> [w323 _]
                              frame False {
                                n166 = Unbundle By Name(w330) -> ("Drive X Position"=w331:dbl)
                                n167 = case shown="False" w328 {
                                tunnel: w331 -> [w334 w336]
                                tunnel: [w333 w337] -> w324
                                tunnel: w323 -> [w332 w335]
                                frame False {
                                n168 = Subtract(x=w334, y=w332) -> (x-y=w333:dbl)
                                }
                                frame True {
                                n169 = Add(x=w336, y=w335) -> (x+y=w337:dbl)
                                }
                                }
                                n170 = Divide(x=w324, y=w323) -> (x/y=w327:dbl)
                                n171 = Round To Nearest(number=w327) -> (nearest integer value=w326:dbl)
                                n172 = Multiply(x=w326, y=w323) -> (x*y=w325:dbl)
                                n173 = Bundle By Name(cluster=w330, "Drive X Position"=w325) -> (w329:T3)
                              }
                              frame True {
                              }
                            }
                            n174 = local write "Target Position"(w316) -> ()
                          }
                          frame #5 {
                            n175 = Tick Count (ms)() -> (millisecond timer value=w343:u32)
                            n176 = Subtract(x=w343, y=w342) -> (x-y=w345:u32)
                            n177 = Divide(x=w345, y=u32 1000) -> (x/y=w340:dbl)
                            n178 = Build Array (concatenate)(w341, w340) -> (w339:dbl[])
                          }
                        }
                        n179 = local read "Start"() -> (w200:bool)
                      }
                    }
                    frame #1 {
                      # "set new Y\nand move to new position"
                      n180 = Increment(x=w357) -> (x+1=w356:i32)
                      n181 = local read "Start"() -> (w347:bool)
                      n182 = Equal?(x=w355, y=w356) -> (x = y?=w349:bool)
                      n183 = local read "Simulate Drive"() -> (w350:bool)
                      n184 = Not(x=w347) -> (.not. x?=w348:bool)
                      n185 = Or(x=w349, y=w348) -> (x .or. y?=w346:bool)
                      n186 = case shown="False" w346 {
                        tunnel: w353 -> [w376 w377]
                        tunnel: [w375 w377] -> w351
                        tunnel: w354 -> [w370 _]
                        frame False {
                          n187 = Unbundle By Name(w376) -> ("Drive Y Position"=w374:dbl)
                          n188 = Add(x=w370, y=w374) -> (x+y=w371:dbl)
                          n189 = Divide(x=w371, y=w370) -> (x/y=w372:dbl)
                          n190 = Round To Nearest(number=w372) -> (nearest integer value=w373:dbl)
                          n191 = Multiply(x=w373, y=w370) -> (x*y=w369:dbl)
                          n192 = Bundle By Name(cluster=w376, "Drive Y Position"=w369) -> (w375:T3)
                        }
                        frame True {
                        }
                      }
                      n193 = case shown="False" w350 {
                        tunnel: w352 -> [w360 _]
                        tunnel: w351 -> [w359 _]
                        frame False {
                          n194 = flat-sequence {
                            tunnel: w360 -> [w365]
                            tunnel: w359 -> [w364]
                            tunnel: [w365] -> w361
                            tunnel: [w368] -> w358
                            tunnel: w361 -> [w367]
                            frame #0 {
                              n195 = Unbundle By Name(w364) -> ("Drive Y Position"=w363:dbl)
                              n196 = control-ref of="Objective Running"() -> (w366:refnum<vi>)
                              n197 = call "NPC3SG Move Axis To.vi"("Drive Visa Name"=w365, "Running"=w366, "Axis"=1, "Drive Set"=w363) -> ()  [unwired: 3 in, 1 out]
                            }
                            frame #1 {
                              n198 = call "NPC3SG Get Values.vi"("Drive Visa Name"=w367) -> ("Drive Current Values"=w368:T3)
                            }
                          }
                          n199 = global write "Global Variables.vi" "Global Piezo Position"(w358) -> ()
                          n200 = local write "Current Position"(w358) -> ()
                        }
                        frame True {
                        }
                      }
                      n201 = local write "Target Position"(w351) -> ()
                    }
                  }
                  n202 = local read "Start"() -> (w143:bool)
                }
              }
              frame #2 {
                # "conclude measurement"
                n203 = flat-sequence {
                  tunnel: w379 -> [w392]
                  tunnel: w378 -> [w391]
                  tunnel: w380 -> [w399]
                  frame #0 {
                    # "save data"
                    n204 = local read "Input Parameters"() -> (w385:T1)
                    n205 = global read "Global Variables.vi" "Global iHR Values"() -> (w388:T4)
                    n206 = global read "Global Variables.vi" "Global ITC Values"() -> (w389:T2)
                    n207 = local read "Spectra Params"() -> (w386:T5)
                    n208 = global read "Global Variables.vi" "Global CCD Temperature (C)"() -> (w387:dbl)
                    n209 = Unbundle By Name(w385) -> ("CCD Area"=w384:T6, "CCD Gain"=w382:u16, "CCD ADC"=w383:u16)
                    n210 = local read "Mapping Params"() -> (w381:T8)
                    n211 = call "Export_mappingFileName v10.5.1.vi"("ITC503 Current Values"=w389, "iHR Current Values"=w388, "Spectra Settings"=w386, "Mapping Parameters"=w381) -> ("Filename"=w395:string)  [unwired: 1 in]
                    "Filename" <- w395
                    n212 = local read "Live Data"() -> (w394:dbl[][])
                    n213 = Unbundle By Name(w381) -> ("Step Size"=w390:dbl)
                    n214 = call "Mapping Merge Real Positions v10.2.1.vi"("Live Data In"=w394, "X in (1D)"=w392, "Y in (1D)"=w391, "Step Size"=w390) -> ("Live Data Out"=w393:dbl[][])  [unwired: 11 in]
                    "Full Data" <- w393
                    n215 = call "Export_2DtoTxt v10.6.0.vi"("ITC503 Current Values"=w389, "iHR Current Values"=w388, "CCD Temperature"=w387, "CCD Area"=w384, "CCD ADC"=w383, "CCD Gain"=w382, "Export Type"="Mapping", "Spectra Settings"=w386, "Filename"=w395, "Data (2D)"=w393, "Mapping Parameters"=w381) -> ()  [unwired: 8 in, 1 out]
                  }
                  frame #1 {
                    # "reset indicators"
                    n216 = case shown="False" w399 {
                      frame False {
                      }
                      frame True {
                      }
                    }
                    n217 = local write "Start"(FALSE ("Start")) -> ()
                    n218 = local write "CCD Current Rep."("0/0" ("CCD3000 Current Rep.")) -> ()
                    n219 = global write "Global Variables.vi" "Mapping Running?"(FALSE ("Mapping Running?")) -> ()
                    n220 = property on="Measuring" class="Bool (strict)"("BoolText.Text"="" ("Boolescher Text.Text")) -> ()  [unwired: 2 in, 2 out]
                    n221 = property on="Measuring" class="Bool (strict)"("Blinking"=FALSE ("Measuring")) -> ()  [unwired: 2 in, 2 out]
                  }
                }
              }
            }
          }
        }
        n222 = local read "Exit"() -> (w40:bool)
      }
    }
    frame #2 {
      n223 = invoke class="VI Interface Type 0" method="Ctrl Val.Set"(reference=w404, "Control Name"="Exit" ("Elementname"), "Value"=TRUE) -> ()  [unwired: 2 in, 5 out]
      n224 = local read "AutoClose"() -> (w403:bool)
      n225 = flat-sequence {
        tunnel: w403 -> [w407]
        frame #0 {
          # "reset and close"
          n226 = control-ref of="Dieses VI"() -> (w410:refnum<vi>)
          n227 = global write "Global Variables.vi" "Mapping Open?"(FALSE ("Mapping Open?")) -> ()
          n228 = invoke class="VI" method="Default Vals.Reinit All"(reference=w410) -> (reference out=w408:refnum<vi>)  [unwired: 2 in, 2 out]
          n229 = property on="Measuring" class="Bool (strict)"("BoolText.Text"="" ("Boolescher Text.Text")) -> ()  [unwired: 2 in, 2 out]
          n230 = property class="App"() -> ("App.Kind"=w411:T12)  [unwired: 2 in, 2 out]
          n231 = case shown="\"Development System\"" w411 {
            tunnel: w408 -> [w413 w415]
            tunnel: w407 -> [_ w414]
            frame "invalid app kind", Default {
              n232 = invoke on="Invoke Node" class="VI" method="FP.Close"(reference=w413) -> ()  [unwired: 2 in, 3 out]
            }
            frame "Development System" {
              n233 = case shown="True" w414 {
                tunnel: w415 -> [_ w416]
                frame False {
                }
                frame True {
                  n234 = invoke on="Invoke Node" class="VI" method="FP.Close"(reference=w416) -> ()  [unwired: 2 in, 3 out]
                }
              }
            }
          }
        }
      }
    }
  }
